vi "Annotation_Rotate.vi"(9 "Rotation":T3, 11 "Annotations (CWH)":T1[](array[typedef]) {"BBox"."x" format="%#_4p"; "BBox"."y" format="%#_4p"; "BBox"."w" format="%#_4p"; "BBox"."h" format="%#_4p"}) -> (3 "Annotations (CWH) out":T1[](array[typedef]) {"BBox"."x" format="%#_4p"; "BBox"."y" format="%#_4p"; "BBox"."w" format="%#_4p"; "BBox"."h" format="%#_4p"})   [LabVIEW 2020]
uses:
  Controls/Aug_Rotation.ctl
  <vilib>/Ngene/Deep Learning Toolkit/Toolkit/NN_Data/API/Data/Detection_Types/NN_BBox_Annotation.ctl
  <vilib>/Ngene/Deep Learning Toolkit/Toolkit/NN_Data/API/Data/Detection_Types/NN_BBox.ctl
  <vilib>/Ngene/Deep Learning Toolkit/Toolkit/NN_Data/API/Data/Detection_Types/NN_BBox_Format_Conversion_Direction.ctl
  <vilib>/Ngene/Deep Learning Toolkit/Toolkit/Deep_Learning_Toolkit_by_Ngene.lvlib
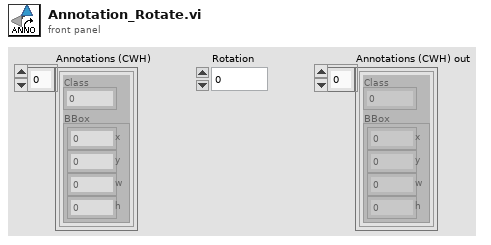
[diagram p1: front panel]
types:
  T1 = typedef "Deep_Learning_Toolkit_by_Ngene.lvlib/NN_BBox_Annotation.ctl" = cluster{"Class":i32, "BBox":T2}
  T2 = typedef "Deep_Learning_Toolkit_by_Ngene.lvlib/NN_BBox.ctl" = cluster{"x":sgl, "y":sgl, "w":sgl, "h":sgl}
  T3 = typedef "Aug_Rotation.ctl" = enum16{"0", "90", "180", "270"}
  T4 = typedef "Deep_Learning_Toolkit_by_Ngene.lvlib/NN_BBox_Format_Conversion_Direction.ctl" = enum16{"SS_to_CWH", "CWH_to_SS"}
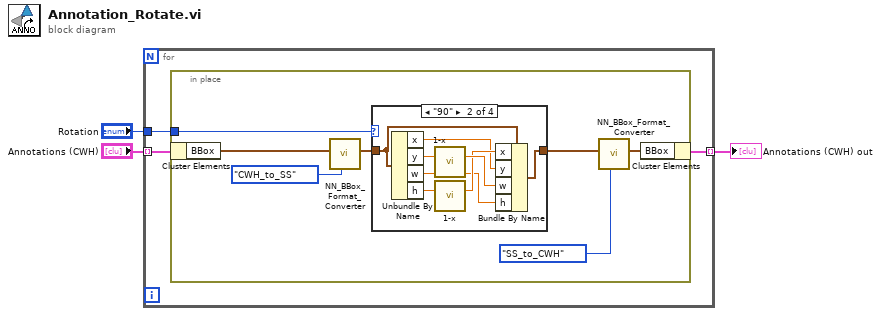
[diagram p0: block diagram]
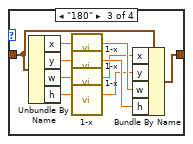
[diagram p3: hidden frame]
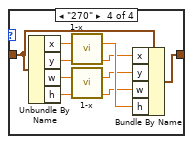
[diagram p4: hidden frame]
diagram:
  n1 = for {
    tunnel: "Annotations (CWH)" -> [w5] mode=indexing
    tunnel: "Rotation" -> [w6]
    tunnel: [w4] -> w2 mode=indexing
    n2 = in-place {
      in-place-border: w6 -> [w13]
      n3 = in-place-cluster #1(w5) -> ("BBox"=w8:T2)
      n4 = call <vilib>:"NN_BBox_Format_Converter.vi"("Conversion_Direction"=NN_BBox_Format_Conversion_Direction."CWH_to_SS" ("Format_Transform"), "BBox in"=w8) -> ("BBox out"=w9:T2)  [unwired: 9 in]
      n5 = case shown="\"90\"" w13 {
        tunnel: w9 -> [w14 w15 w32 w33]
        tunnel: [w14 w20 w31 w38] -> w10
        frame "0", Default {
        }
        frame "90" {
          n6 = Unbundle By Name(w15) -> ("x"=w19:sgl, "y"=w18:sgl, "w"=w17:sgl, "h"=w16:sgl)
          n7 = call "1-x.vi"("x"=w18) -> ("1-x"=w22:sgl)  [unwired: 14 in]
          n8 = call "1-x.vi"("x"=w16) -> ("1-x"=w21:sgl)  [unwired: 14 in]
          n9 = Bundle By Name(cluster=w15, "x"=w21, "y"=w19, "w"=w22, "h"=w17) -> (w20:T2)
        }
        frame "180" {
          n10 = Unbundle By Name(w32) -> ("x"=w30:sgl, "y"=w29:sgl, "w"=w28:sgl, "h"=w27:sgl)
          n11 = call "1-x.vi"("x"=w30) -> ("1-x"=w26:sgl)  [unwired: 14 in]
          n12 = call "1-x.vi"("x"=w29) -> ("1-x"=w25:sgl)  [unwired: 14 in]
          n13 = call "1-x.vi"("x"=w28) -> ("1-x"=w24:sgl)  [unwired: 14 in]
          n14 = call "1-x.vi"("x"=w27) -> ("1-x"=w23:sgl)  [unwired: 14 in]
          n15 = Bundle By Name(cluster=w32, "x"=w24, "y"=w23, "w"=w26, "h"=w25) -> (w31:T2)
        }
        frame "270" {
          n16 = Unbundle By Name(w33) -> ("x"=w37:sgl, "y"=w36:sgl, "w"=w35:sgl, "h"=w34:sgl)
          n17 = call "1-x.vi"("x"=w37) -> ("1-x"=w40:sgl)  [unwired: 14 in]
          n18 = call "1-x.vi"("x"=w35) -> ("1-x"=w39:sgl)  [unwired: 14 in]
          n19 = Bundle By Name(cluster=w33, "x"=w36, "y"=w39, "w"=w34, "h"=w40) -> (w38:T2)
        }
      }
      n20 = call <vilib>:"NN_BBox_Format_Converter.vi"("Conversion_Direction"=NN_BBox_Format_Conversion_Direction."SS_to_CWH" ("Format_Transform"), "BBox in"=w10) -> ("BBox out"=w7:T2)  [unwired: 9 in]
      n21 = in-place-cluster #1("BBox"=w7) -> (w4:T1)
    }
  }
  "Annotations (CWH) out" <- w2
